vi "FinalSerial.vi"() -> ()   [LabVIEW 2020]
panel:
  in  "stop":bool
  out "Lectura":string
  in  "Serial":enum32{"DashBoard", "Grafos", "Configuracion"}(tab)
  out "Voltaje":dbl[](array[slide]) scale=0.0..5.0
  in  "LED 4":bool
  in  "LED 3":bool
  in  "LED 2":bool
  in  "LED 1":bool
  out "ADC":i32[](array[slide]) scale=0.0..1023.0
  out "In Digital":i32[](array[numeric])
  out "Waveform Chart 2":cluster{dbl, dbl}(graph)
  out "Waveform Chart":cluster{dbl, dbl}(graph)
  in  "Serial Init":T1={"Puerto Serial"="", "baud rate (9600)"=9600, "data bits (8)"=8, "parity (0:none)"=enum."None", "error in (no error)"={"status"=FALSE, "code"=0, "source"=""}, "stop bits (10: 1 bit)"=10, "flow control (0:none)"=0} {"flow control (0:none)" items=["None", "XON/XOFF", "RTS/CTS", "XON/XOFF & RTS/CTS", "DTR/DSR", "XON/XOFF & DTR/DSR"]; "stop bits (10: 1 bit)" items=["1.0"=10, "1.5"=15, "2.0"=20]; "data bits (8)" min=5 max=8 step=1}
  # "Serial Final"
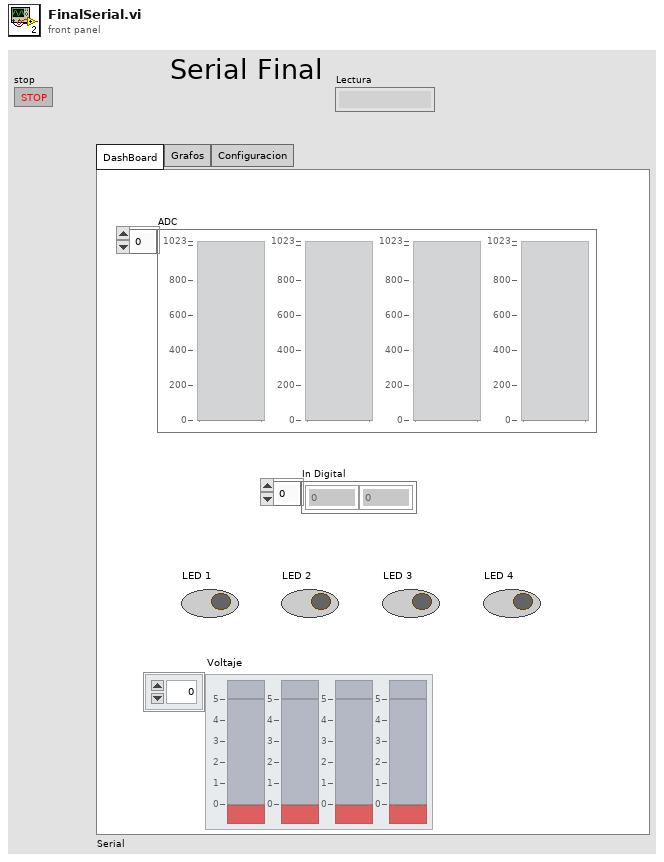
[diagram p1: front panel]
types:
  T1 = cluster{"Puerto Serial":refnum<visa-resource-name>, "baud rate (9600)":u32, "data bits (8)":u16, "parity (0:none)":enum16{"None", "Odd", "Even", "Mark", "Space"}, "error in (no error)":errorcluster, "stop bits (10: 1 bit)":u16, "flow control (0:none)":u16}
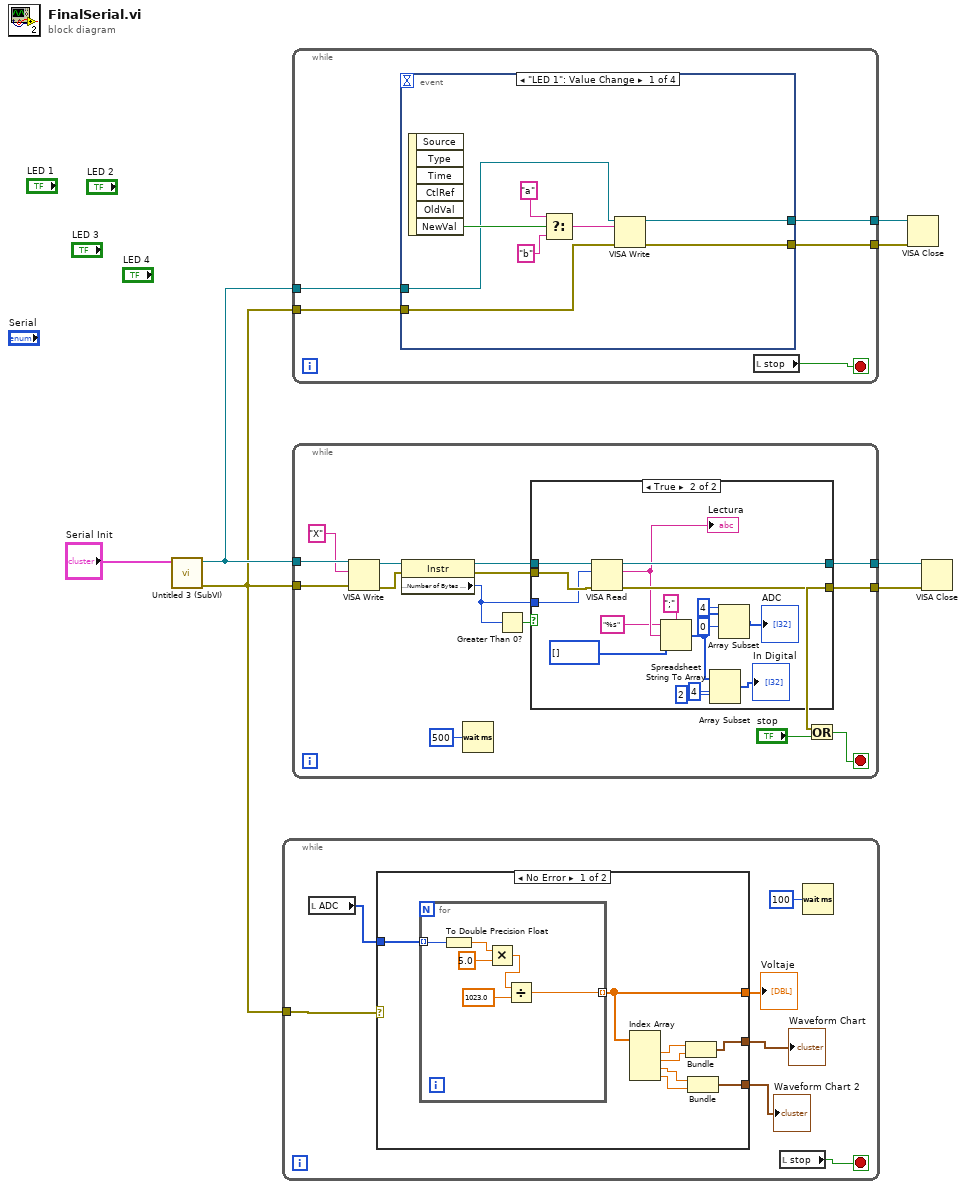
[diagram p0: block diagram]
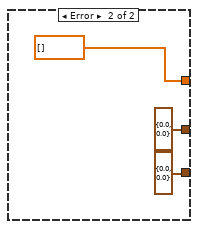
[diagram p2: hidden frame]
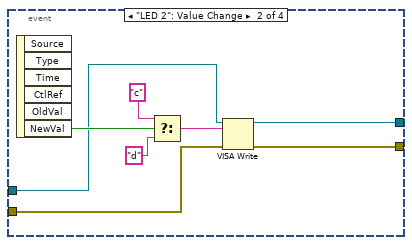
[diagram p4: hidden frame]
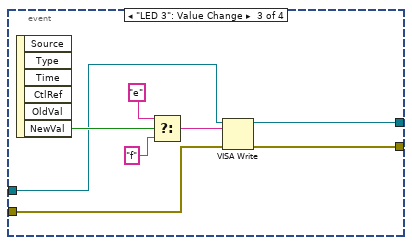
[diagram p5: hidden frame]
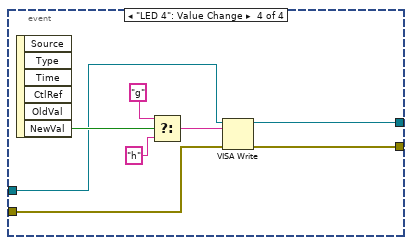
[diagram p6: hidden frame]
diagram:
  n1 = call "Untitled 3 (SubVI).vi"("Serial Init"="Serial Init") -> ("error out"=w1:errorcluster, "VISA Refnum out"=w4:refnum<visa-resource-name>)  [unwired: 9 in]
  n2 = while {
    tunnel: w1 -> [w13]
    stop <- w14 stop-if-true
    n3 = local read "ADC"() -> (w12:i32[])
    n4 = case shown="No Error" w13 {
      tunnel: w12 -> [w22 _]
      tunnel: [w21 dbl[] []] -> w11
      tunnel: [w16 cluster{dbl, dbl} {0.0, 0.0}] -> w10
      tunnel: [w15 cluster{dbl, dbl} {0.0, 0.0}] -> w9
      frame No Error {
        n5 = for {
          tunnel: w22 -> [w23] mode=indexing
          tunnel: [w24] -> w21 mode=indexing
          n6 = To Double Precision Float(number=w23) -> (double precision float=w28:dbl)
          n7 = Multiply(x=w28, y=5.0) -> (x*y=w27:dbl)
          n8 = Divide(x=w27, y=1023.0) -> (x/y=w24:dbl)
        }
        n9 = Index Array(array=w21) -> (element #1=w20:dbl, element #2=w19:dbl, element #3=w17:dbl, element #4=w18:dbl)  [unwired: 4 in]
        n10 = Bundle(w20, w19) -> (w15:cluster{dbl, dbl})  [unwired: 1 in]
        n11 = Bundle(w17, w18) -> (w16:cluster{dbl, dbl})  [unwired: 1 in]
      }
      frame Error {
      }
    }
    "Voltaje" <- w11
    "Waveform Chart" <- w9
    "Waveform Chart 2" <- w10
    n12 = local read "stop"() -> (w14:bool)
    n13 = Wait (ms)(milliseconds to wait=u32 100) -> ()  [unwired: 1 out]
  }
  n14 = while {
    tunnel: w4 -> [w36]
    tunnel: w1 -> [w35]
    tunnel: [w34] -> w3
    tunnel: [w33] -> w2
    stop <- w32 stop-if-true
    n15 = event shown="[0] \"LED 1\": Value Change" {
      selector: _ -> [_ _ _ _]
      dyn-events: _ -> [_ _ _ _]
      timeout: _ -> [_ _ _ _]
      tunnel: w36 -> [w40 w48 w56 w64]
      tunnel: w35 -> [w39 w47 w55 w63]
      tunnel: [w38 w46 w54 w62] -> w34
      tunnel: [w37 w45 w53 w61] -> w33
      event "LED 1": Value Change {
        n16 = event-data() -> ("NewVal"=w44:bool)  [unwired: 1 in, 5 out]
        n17 = Select(t="a", s=w44, f="b") -> (s? t:f=w41:string)
        n18 = VISA Write(VISA resource name=w40, write buffer=w41, error in (no error)=w39) -> (VISA resource name out=w38:refnum<visa-resource-name>, error out=w37:errorcluster)  [unwired: 1 out]
      }
      event "LED 2": Value Change {
        n19 = event-data() -> ("NewVal"=w52:bool)  [unwired: 1 in, 5 out]
        n20 = Select(t="c", s=w52, f="d") -> (s? t:f=w49:string)
        n21 = VISA Write(VISA resource name=w48, write buffer=w49, error in (no error)=w47) -> (VISA resource name out=w46:refnum<visa-resource-name>, error out=w45:errorcluster)  [unwired: 1 out]
      }
      event "LED 3": Value Change {
        n22 = event-data() -> ("NewVal"=w60:bool)  [unwired: 1 in, 5 out]
        n23 = Select(t="e", s=w60, f="f") -> (s? t:f=w57:string)
        n24 = VISA Write(VISA resource name=w56, write buffer=w57, error in (no error)=w55) -> (VISA resource name out=w54:refnum<visa-resource-name>, error out=w53:errorcluster)  [unwired: 1 out]
      }
      event "LED 4": Value Change {
        n25 = event-data() -> ("NewVal"=w68:bool)  [unwired: 1 in, 5 out]
        n26 = Select(t="g", s=w68, f="h") -> (s? t:f=w65:string)
        n27 = VISA Write(VISA resource name=w64, write buffer=w65, error in (no error)=w63) -> (VISA resource name out=w62:refnum<visa-resource-name>, error out=w61:errorcluster)  [unwired: 1 out]
      }
    }
    n28 = local read "stop"() -> (w32:bool)
  }
  n29 = while {
    tunnel: w4 -> [w82]
    tunnel: w1 -> [w81]
    tunnel: [w74] -> w6
    tunnel: [w70] -> w5
    stop <- w71 stop-if-true
    n30 = VISA Write(VISA resource name=w82, write buffer="X", error in (no error)=w81) -> (VISA resource name out=w79:refnum<visa-resource-name>, error out=w78:errorcluster)  [unwired: 1 out]
    n31 = property class="Instr"(reference=w79, error in=w78) -> (reference out=w76:refnum<visa-resource-name>, error out=w75:errorcluster, "Serial Settings:Number of Bytes at Serial Port"=w73:u32)
    n32 = Wait (ms)(milliseconds to wait=u32 500) -> ()  [unwired: 1 out]
    n33 = Greater Than 0?(x=w73) -> (x > 0?=w77:bool)
    n34 = case shown="True" w77 {
      tunnel: w76 -> [w84 w100]
      tunnel: w75 -> [w83 w99]
      tunnel: [w84 w97] -> w74
      tunnel: [w83 w96] -> w70
      tunnel: w73 -> [_ w98]
      frame False {
      }
      frame True {
        n35 = VISA Read(VISA resource name=w100, byte count=w98, error in (no error)=w99) -> (VISA resource name out=w97:refnum<visa-resource-name>, read buffer=w94:string, error out=w96:errorcluster)  [unwired: 1 out]
        "Lectura" <- w94
        n36 = Spreadsheet String To Array(delimiter (Tab)=";", format string="%s", spreadsheet string=w94, array type (2D Dbl)=i32[] []) -> (array=w90:i32[])
        n37 = Array Subset(array=w90, index=4, length=2) -> (→"In Digital":i32[])
        n38 = Array Subset(array=w90, index=0, length=4) -> (→"ADC":i32[])
      }
    }
    n39 = Or(x=w70, y="stop") -> (x .or. y?=w71:bool)
  }
  n40 = VISA Close(VISA resource name=w3, error in (no error)=w2) -> ()  [unwired: 1 out]
  n41 = VISA Close(VISA resource name=w6, error in (no error)=w5) -> ()  [unwired: 1 out]
